vi "EasyXML Options - Flatten Data.vi"(8 "error in":errorcluster, 11 "Easy XML Options in":T1) -> (0 "error out":errorcluster, 3 "EasyXML Options out":T4)   [LabVIEW 2011]
uses:
  Support/Type Defs/EasyXML Options.ctl
  EasyXML Options - Data Cluster.ctl
  EasyXML Options - Type Formatting Cluster.ctl
  Support/Type Defs/Formatting Data Type -- Enum.ctl
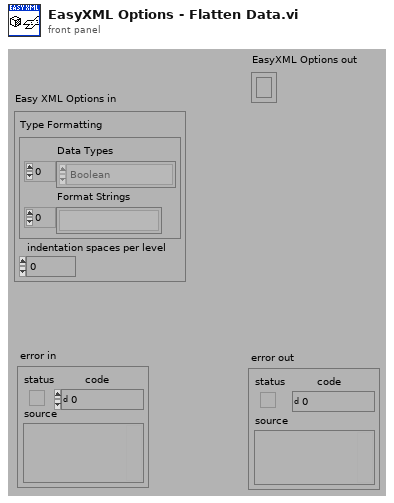
[diagram p1: front panel]
types:
  T1 = typedef "EasyXML Options - Data Cluster.ctl" = cluster{"Type Formatting":T2, "indentation spaces per level":i32}
  T2 = typedef "EasyXML Options - Type Formatting Cluster.ctl" = cluster{"Data Types":T3[], "Format Strings":string[]}
  T3 = typedef "Formatting Data Type -- Enum.ctl" = enum16{"<unknown>", "Cluster", "Array", "String", "Path", "Boolean", "Time Stamp", "Enum", "Numeric - EXT", "Numeric - DBL", "Numeric - SGL", "Numeric - I64", "Numeric - I32", "Numeric - I16", "Numeric - I8", "Numeric - U64", "Numeric - U32", "Numeric - U16", "Numeric - U8", "Numeric - CXT", "Numeric - CDB", "Numeric - CSG", "VISA Resource"}
  T4 = typedef "EasyXML Options.ctl" = cluster{"Data":variant}
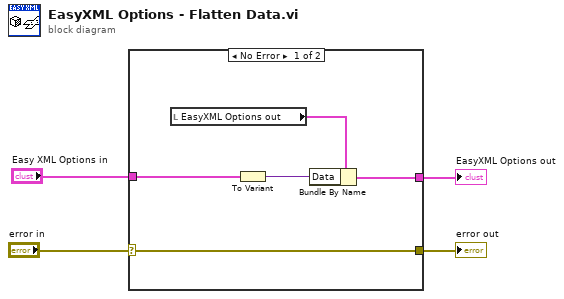
[diagram p0: block diagram]
diagram:
  n1 = case shown="No Error" "error in" {
    selector: "error in" -> [w8 w10]
    tunnel: "Easy XML Options in" -> [w9 _]
    tunnel: [w8 w10] -> w4
    tunnel: [w5 _] -> w1
    frame No Error {
      n2 = local read "EasyXML Options out"() -> (w7:T4)
      n3 = To Variant(anything=w9) -> (Variant=w6:variant)
      n4 = Bundle By Name(cluster=w7, "Data"=w6) -> (w5:T4)
    }
    frame Error {
    }
  }
  "EasyXML Options out" <- w1
  "error out" <- w4
